vi "Configure Math (Unary Operation).vi"(0 "VISA resource name":refnum<visa-resource-name>, 1 "Enable Math Channel (T:Enable)":bool, 2 "# of Averages (16)":i32, 3 "FFTWindow (0:Rectangular)":u16(ring) items=["Rectangular", "Hanning", "FlatTop"], 5 "Math Channel (5: Function 1)":i32(ring) items=["Function 1", "Function 2", "Function 3", "Function 4"], 7 "Math Operand (1: Channel 1)":i32(ring) items=["Channel 1", "Channel 2", "Channel 3", "Channel 4", "Function 1", "Function 2", "Function 3", "Function 4", "Memory 1", "Memory 2", "Memory 3", "Memory 4"], 9 "Math Operation (0: Average)":u16(ring) items=["Average", "Differentiate", "FFT Magnitude", "FFT Phase", "High Pass Filter", "Integrate", "Invert", "Low Pass Filter", "Magnify", "Max", "Min", "Smooth"], 11 "error in (no error)":errorcluster, 12 "Bandwidth (350E6)":dbl, 13 "Smoothing Points (5)":i32) -> (4 "VISA resource name out":refnum<visa-resource-name>, 15 "error out":errorcluster)   [LabVIEW 2009, in "Agilent 8000 Series.lvlib"]
doc: "Creates a mathematical expression with one operand."
uses:
  Agilent 8000 Series.lvlib
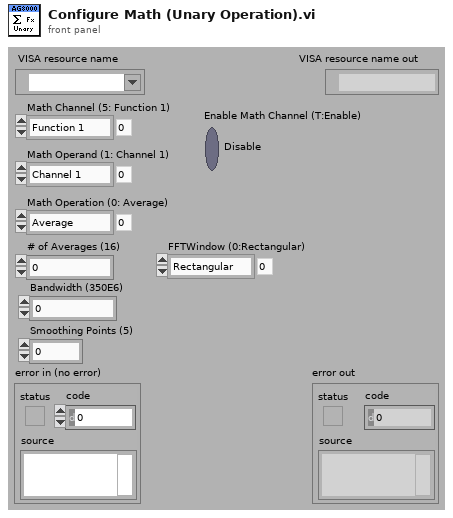
[diagram p1: front panel]
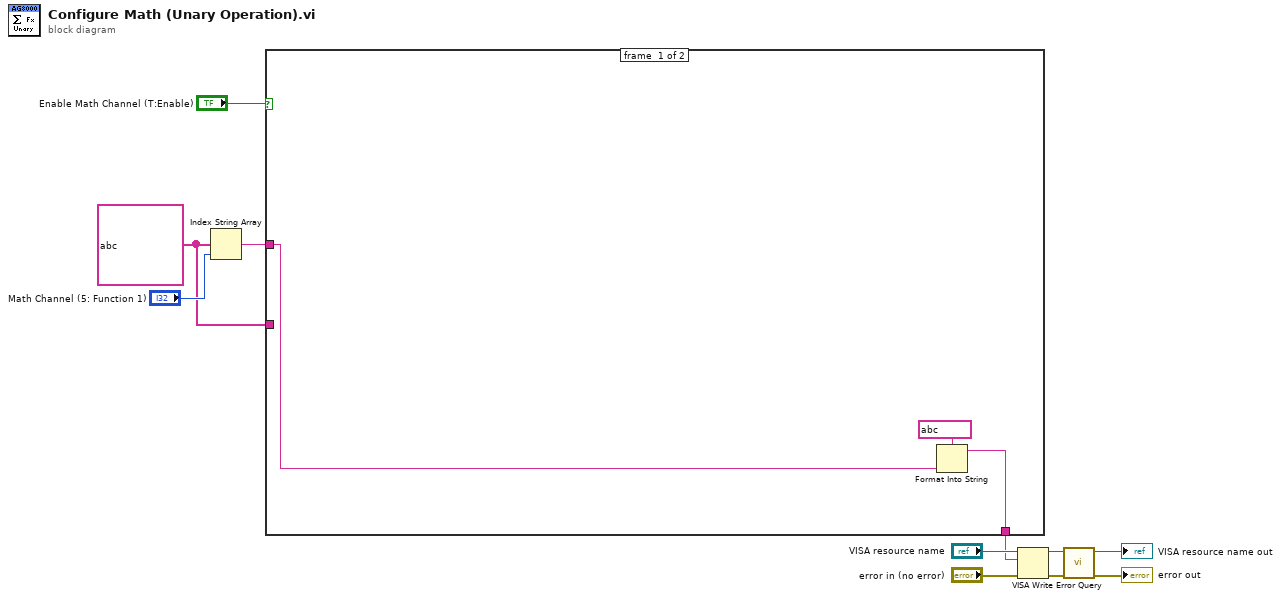
[diagram p0: block diagram]
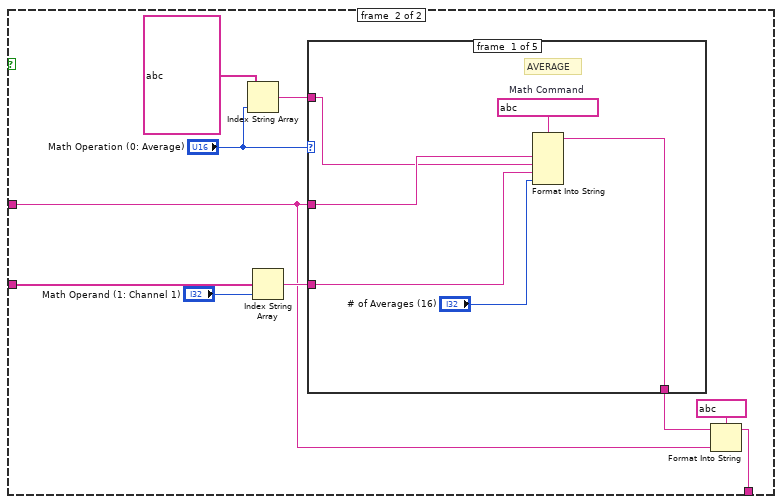
[diagram p2: hidden frame]
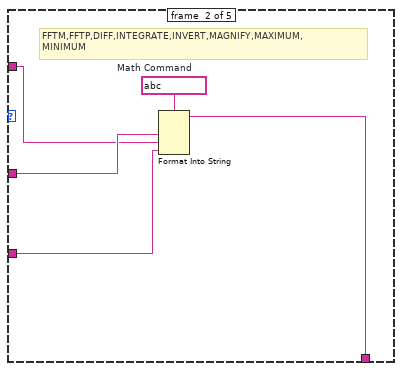
[diagram p3: hidden frame]
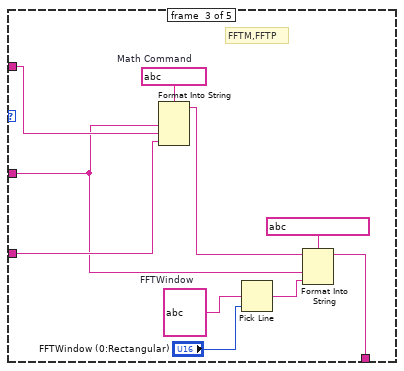
[diagram p4: hidden frame]
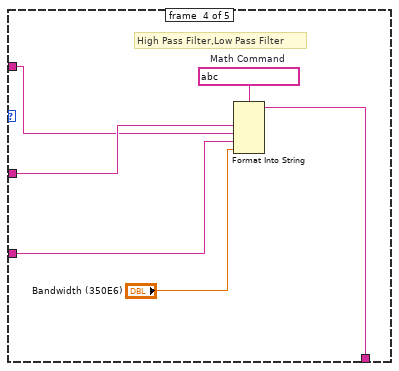
[diagram p5: hidden frame]
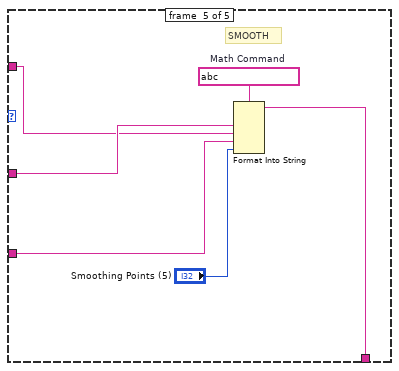
[diagram p6: hidden frame]
diagram:
  w3 = string[] ?
  n1 = Index String Array(1:"Math Channel (5: Function 1)", 2:w3) -> (0:w4:string)  [unwired: 1 in]
  n2 = case shown="True" "Enable Math Channel (T:Enable)" {
    tunnel: w4 -> [w13 w16]
    tunnel: w3 -> [_ w20]
    tunnel: [w12 w15] -> w1
    frame #0 {
      n3 = Format Into String(format string=string ?, w13) -> (resulting string=w12:string)  [unwired: 2 in, 1 out]
    }
    frame #1 {
      n4 = Index String Array(1:"Math Operation (0: Average)", 2:string[] ?) -> (0:w22:string)  [unwired: 1 in]
      n5 = Index String Array(1:"Math Operand (1: Channel 1)", 2:w20) -> (0:w19:string)  [unwired: 1 in]
      n6 = case shown="11" "Math Operation (0: Average)" {
        tunnel: w16 -> [w30 w35 w37 w51 w57]
        tunnel: w22 -> [w29 w34 w45 w50 w56]
        tunnel: w19 -> [w28 w33 w44 w49 w55]
        tunnel: [w25 w31 w36 w46 w52] -> w18
        frame #0 {
          w27 = string ?  # Math Command
          # "AVERAGE"
          n7 = Format Into String(format string=w27, w30, w29, w28, "# of Averages (16)") -> (resulting string=w25:string)  [unwired: 2 in, 1 out]
        }
        frame #1 {
          w32 = string ?  # Math Command
          # "FFTM,FFTP,DIFF,INTEGRATE,INVERT,MAGNIFY,MAXIMUM,\nMINIMUM"
          n8 = Format Into String(format string=w32, w35, w34, w33) -> (resulting string=w31:string)  [unwired: 2 in, 1 out]
        }
        frame #2 {
          w42 = string ?  # FFTWindow
          w43 = string ?  # Math Command
          # "FFTM,FFTP"
          n9 = Format Into String(format string=w43, w37, w45, w44) -> (resulting string=w39:string)  [unwired: 2 in, 1 out]
          n10 = Pick Line(multi-line string=w42, line index="FFTWindow (0:Rectangular)") -> (output string=w38:string)  [unwired: 1 in]
          n11 = Format Into String(format string=string ?, initial string=w39, w37, w38) -> (resulting string=w36:string)  [unwired: 1 in, 1 out]
        }
        frame #3 {
          w48 = string ?  # Math Command
          # "High Pass Filter,Low Pass Filter"
          n12 = Format Into String(format string=w48, w51, w50, w49, "Bandwidth (350E6)") -> (resulting string=w46:string)  [unwired: 2 in, 1 out]
        }
        frame #4 {
          w54 = string ?  # Math Command
          # "SMOOTH"
          n13 = Format Into String(format string=w54, w57, w56, w55, "Smoothing Points (5)") -> (resulting string=w52:string)  [unwired: 2 in, 1 out]
        }
      }
      n14 = Format Into String(format string=string ?, initial string=w18, w16) -> (resulting string=w15:string)  [unwired: 1 in, 1 out]
    }
  }
  n15 = VISA Write(VISA resource name="VISA resource name", write buffer=w1, error in (no error)="error in (no error)") -> (VISA resource name out=w7:refnum<visa-resource-name>, error out=w6:errorcluster)  [unwired: 1 out]
  n16 = call "Error Query.vi"("error in (no error)"=w6, "VISA resource name"=w7) -> ("error out"=→"error out":errorcluster, "VISA resource name out"=→"VISA resource name out":refnum<visa-resource-name>)  [unwired: 6 in, 2 out]
